vi "strip_string.vi"(9 "end":string, 10 "begin":string, 11 "string":string) -> (3 "stripped string":string)   [LabVIEW 2019, in "State Machine API.lvlib"]
uses:
  State Machine API.lvlib
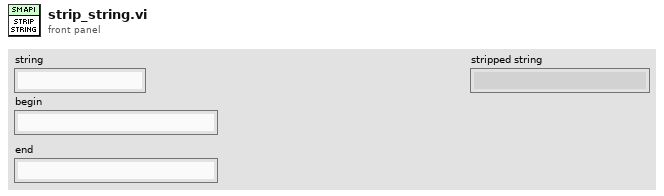
[diagram p1: front panel]
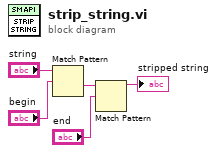
[diagram p0: block diagram]
diagram:
  n1 = Match Pattern(string="string", regular expression="begin") -> (after substring=w3:string)  [unwired: 1 in, 3 out]
  n2 = Match Pattern(string=w3, regular expression="end") -> (before substring=→"stripped string":string)  [unwired: 1 in, 3 out]
